vi "stage_move_axis_relative.vi"(3 "Achse":i32, 5 "Schrittweite [µm]":dbl) -> (0 "error out":errorcluster, 1 "Fertig?":bool, 2 "xyz-Position OUT [mm]":dbl[](array[numeric]))   [LabVIEW 2009]
panel:
  out "Fahren?":bool
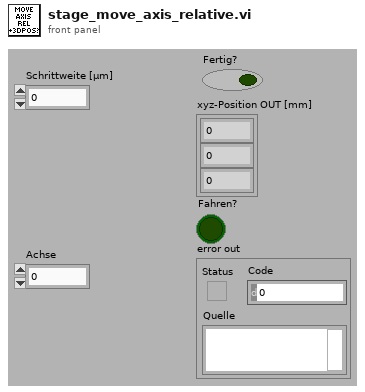
[diagram p1: front panel]
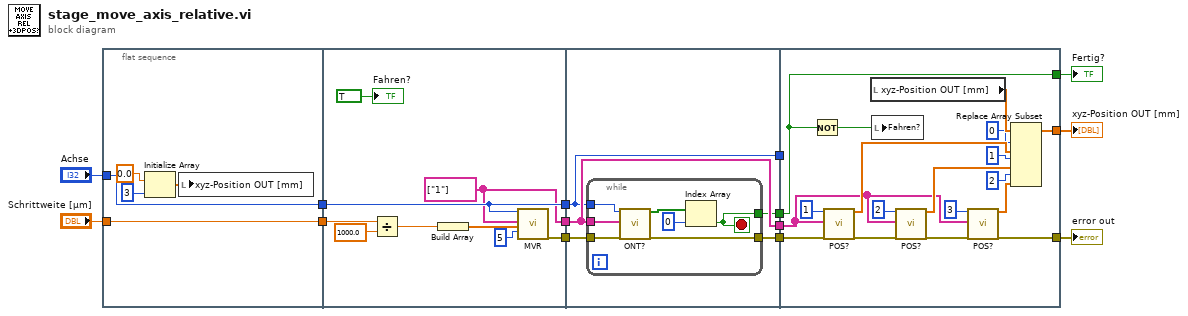
[diagram p0: block diagram]
diagram:
  n1 = flat-sequence {
    tunnel: "Schrittweite [µm]" -> [w18]
    tunnel: "Achse" -> [w19]
    tunnel: [w19] -> w4
    tunnel: [w18] -> w3
    tunnel: [w23] -> w12
    tunnel: [w22] -> w9
    tunnel: [w21] -> w6
    tunnel: w4 -> [w22]
    tunnel: w3 -> [w28]
    tunnel: w12 -> [w33]
    tunnel: [w32] -> w11
    tunnel: w9 -> [w30]
    tunnel: [w30] -> w8
    tunnel: w6 -> [w31]
    tunnel: [w31] -> w5
    tunnel: [w29] -> w2
    tunnel: w11 -> [w58]
    tunnel: [w52] -> w10
    tunnel: w8 -> [_]
    tunnel: [w56] -> w7
    tunnel: w5 -> [w43]
    tunnel: w2 -> [w41]
    tunnel: [w41] -> w1
    frame #0 {
      n2 = Initialize Array(0.0 ("Element"), 3 ("Dimension")) -> (w17:dbl[])
      n3 = local write "xyz-Position OUT [mm]"(w17) -> ()
    }
    frame #1 {
      w21 = string[] ["1"] ("Axes to move")
      n4 = Divide(x=w28, y=1000.0) -> (x/y=w25:dbl)
      n5 = Build Array(w25) -> (w27:dbl[])
      n6 = call "MVR.vi"("System no."=w22, "Axes to move"=w21, "Position values"=w27, "No.of digits"=i16 5) -> ("error out"=w23:errorcluster)  [unwired: 15 in]
      "Fahren?" <- TRUE ("Fahren?")
    }
    frame #2 {
      n7 = while {
        tunnel: w33 -> [w40]
        tunnel: [w39] -> w32
        tunnel: w31 -> [w38]
        tunnel: w30 -> [w37]
        tunnel: [w34] -> w29
        stop <- w34 stop-if-true
        n8 = call "ONT?.vi"("System no."=w37, "Axes to query"=w38, "error in"=w40) -> ("Axis on target?"=w35:bool[], "error out"=w39:errorcluster)  [unwired: 15 in]
        n9 = Index Array(array=w35, index=0 ("Index")) -> (element=w34:bool)
      }
    }
    frame #3 {
      n10 = Not(x=w41) -> (.not. x?=w42:bool)
      n11 = call "POS?.vi"("System no."=1, "Axes to query"=w43, "error in"=w58) -> ("Position"=w57:dbl[], "error out"=w54:errorcluster)  [unwired: 15 in]
      n12 = local read "xyz-Position OUT [mm]"() -> (w55:dbl[])
      n13 = local write "Fahren?"(w42) -> ()
      n14 = call "POS?.vi"("System no."=2, "Axes to query"=w43, "error in"=w54) -> ("Position"=w45:dbl[], "error out"=w53:errorcluster)  [unwired: 15 in]
      n15 = call "POS?.vi"("System no."=3, "Axes to query"=w43, "error in"=w53) -> ("Position"=w44:dbl[], "error out"=w52:errorcluster)  [unwired: 15 in]
      n16 = Replace Array Subset(array=w55, new element #1=w57, index #1=0 ("Index"), new element #2=w45, index #2=1 ("Index"), new element #3=w44, index #3=2 ("Index")) -> (w56:dbl[])
    }
  }
  "Fertig?" <- w1
  "xyz-Position OUT [mm]" <- w7
  "error out" <- w10
